vi "_reportError.vi"(8 "error in (no error)":errorcluster, 11 "SkynetCompiler in":refnum<class "LVAutomationListener.lvclass">) -> (0 "error out":errorcluster, 2 "Error Text":string, 3 "SkynetCompiler out":refnum<class "LVAutomationListener.lvclass">)   [LabVIEW 2013, in "LVAutomationListener.lvlib" / "LVAutomationListener.lvclass"]
doc: "VI puts error message in an error file. This file is used by the make file to report the error to the user."
uses:
  LVAutomationListener.lvclass
  <vilib>/Utility/error.llb/DialogType.ctl
  LVAutomationListener.lvclass/LVAutomationListener.ctl
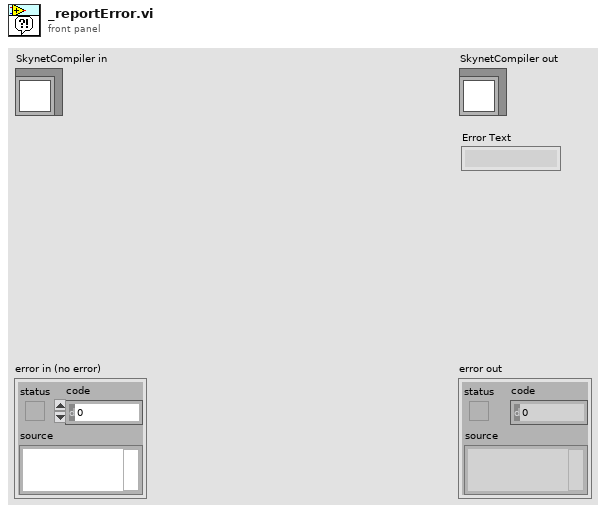
[diagram p1: front panel]
types:
  T1 = enum16{"open", "replace", "create", "open or create", "replace or create", "replace or create with confirmation"}
  T2 = typedef "DialogType.ctl" = u16
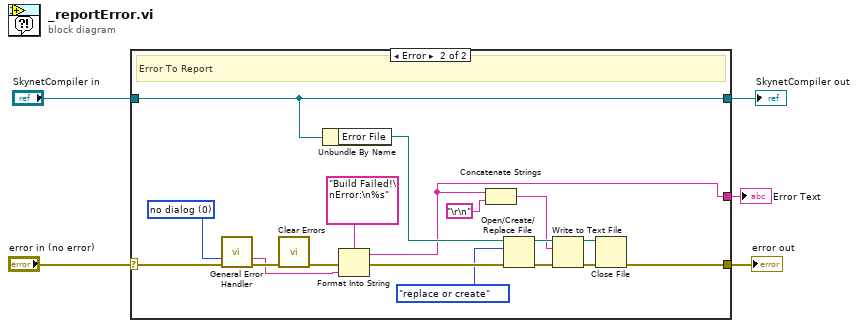
[diagram p0: block diagram]
diagram:
  n1 = case shown="Error" "error in (no error)" {
    selector: "error in (no error)" -> [w6 w25]
    tunnel: [w6 w10] -> w4
    tunnel: [w7 w18] -> w2
    tunnel: "SkynetCompiler in" -> [w7 w18]
    tunnel: [_ w8] -> w1
    frame No Error {
      # "No Error to Report Just Return"
    }
    frame Error {
      w24 = T2 0 items=["no dialog", "OK message", "continue or stop message", "OK message + warnings", "continue/stop + warnings"] ("type of dialog (OK msg:1)")
      # "Error To Report"
      n2 = call <vilib>:"General Error Handler.vi"("type of dialog (OK msg:1)"=w24, "error in (no error)"=w25) -> ("message"=w20:string, "error out"=w23:errorcluster)  [unwired: 9 in, 3 out]
      n3 = call <vilib>:"Clear Errors.vi"("error in (no error)"=w23) -> ("error out"=w22:errorcluster)  [unwired: 6 in]
      n4 = Unbundle By Name(w18) -> ("Error File"=w17:path)
      n5 = Format Into String(format string="Build Failed!\nError:\n%s", error in=w22, w20) -> (resulting string=w8:string, error out=w19:errorcluster)  [unwired: 1 in]
      n6 = Concatenate Strings(w8, "\r\n") -> (w9:string)
      n7 = Open/Create/Replace File(file path (use dialog)=w17, error in=w19, operation (0:open)=T1."replace or create") -> (refnum out=w13:refnum<file>, error out=w15:errorcluster)  [unwired: 3 in, 1 out]
      n8 = Write to Text File(file (use dialog)=w13, text=w9, error in=w15) -> (refnum out=w12:refnum<file>, error out=w11:errorcluster)  [unwired: 1 in, 1 out]
      n9 = Close File(refnum=w12, error in=w11) -> (error out=w10:errorcluster)  [unwired: 1 out]
    }
  }
  "error out" <- w4
  "SkynetCompiler out" <- w2
  "Error Text" <- w1
